vi "BLE_Sample - Test1.vi"() -> (2 "Table Control":string[][](table))   [LabVIEW 2020]
uses:
  C:/Users/bharathi.t/Downloads/Bluetooth - Copy/Bluetooth/BLE/BLELib.dll
  BLELib.dll
panel:
  out "DisConnect_BLE_ByAddress":bool
  out "ConnectionStatusChanged":string
  out "Numeric 2":i32
  out "error out":errorcluster
  out "Pair Result":string
  # "A4:DA:32:0D:F5:E2"
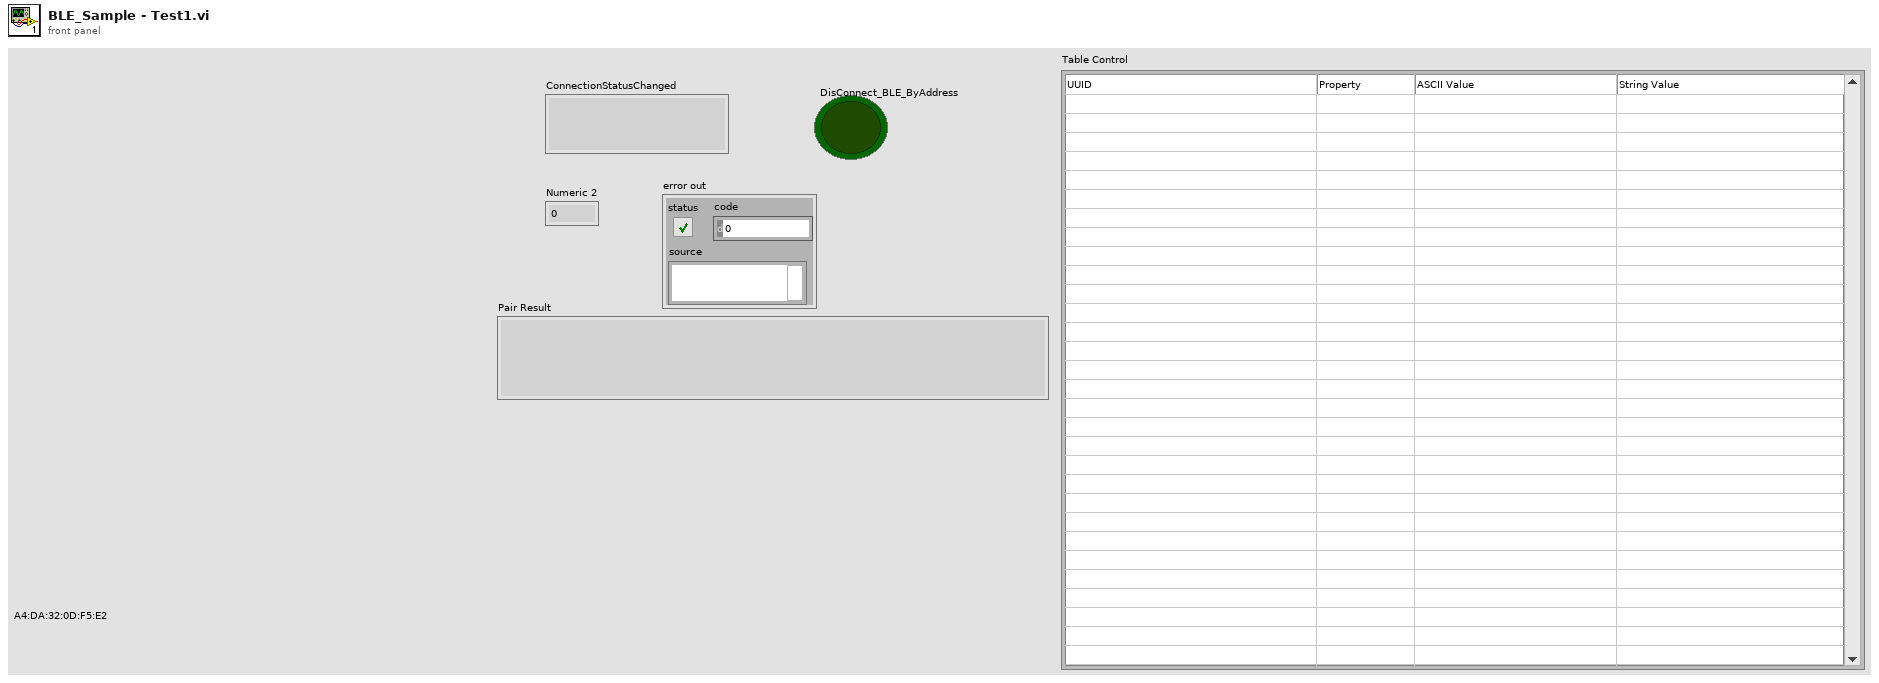
[diagram p1: front panel]
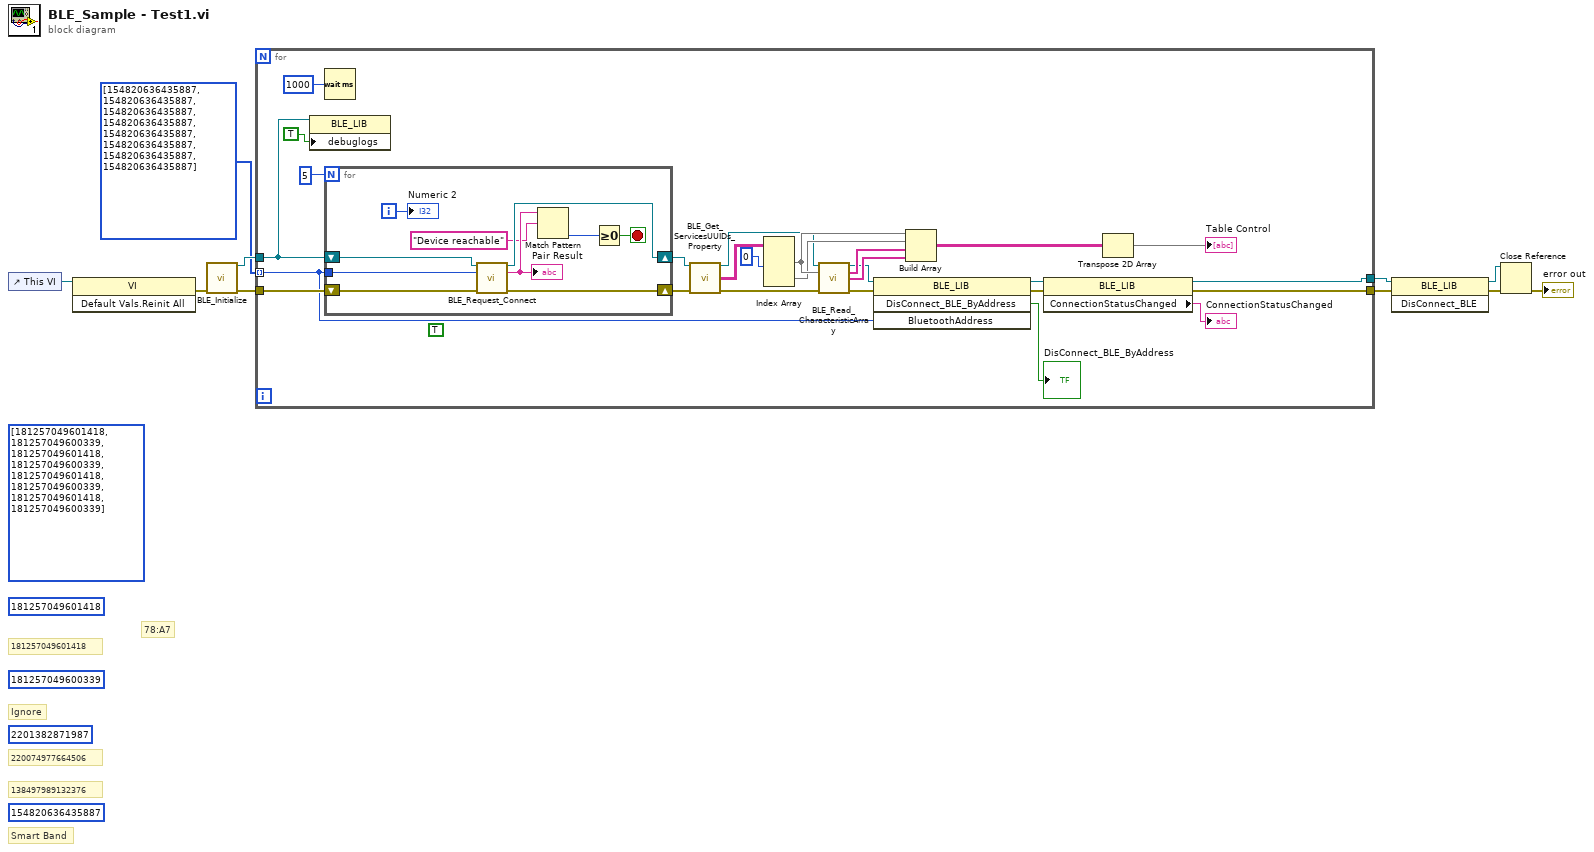
[diagram p0: block diagram]
diagram:
  (unwired) u64[] [181257049601418, 181257049600339, 181257049601418, 181257049600339, 181257049601418, 181257049600339, 181257049601418, 181257049600339]
  (unwired) u64 181257049600339 ("BluetoothAddress")
  (unwired) u64 2201382871987 ("BluetoothAddress")
  (unwired) u64 154820636435887 ("BluetoothAddress")
  (unwired) u64 181257049601418 ("BluetoothAddress")
  # "138497989132376"
  # "220074977664506"
  # "Ignore"
  # "78:A7"
  # "181257049601418"
  # "Smart Band"
  n1 = control-ref of="This VI"() -> (w10:refnum<vi>)
  n2 = invoke class="VI" method="Default Vals.Reinit All"(reference=w10) -> (error out=w8:errorcluster)  [unwired: 2 in, 2 out]
  n3 = call "BLE_Initialize.vi"("error in (no error)"=w8) -> (".NET Refnum out"=w6:refnum<k24>, "error out"=w7:errorcluster)  [unwired: 13 in]
  n4 = for {
    tunnel: [w14] -> w4
    tunnel: w6 -> [w21]
    tunnel: w7 -> [w20]
    tunnel: u64[] [154820636435887, 154820636435887, 154820636435887, 154820636435887, 154820636435887, 154820636435887, 154820636435887, 154820636435887] -> [w17] mode=indexing
    tunnel: [w15] -> w2
    (unwired) TRUE
    n5 = property class="BLE_LIB"(reference=w21, "debuglogs"=TRUE) -> ()  [unwired: 1 in, 2 out]
    n6 = Wait (ms)(milliseconds to wait=u32 1000) -> ()  [unwired: 1 out]
    n7 = for {
      N: 5 -> [_]
      tunnel: w17 -> [w44]
      shift-right: [w42] -> w34
      shift-left: w20 -> [w46]
      shift-right: [w43] -> w35
      shift-left: w21 -> [w45]
      i -> [w37]
      stop <- w38 stop-if-true
      n8 = call "BLE_Request_Connect.vi"(".NET Refnum in"=w45, "BluetoothAddress"=w44, "error in (no error)"=w46) -> (".NET Refnum out"=w43:refnum<k24>, "ConnectBLE"=w41:string, "error out"=w42:errorcluster)  [unwired: 10 in]
      "Pair Result" <- w41
      n9 = Match Pattern(string=w41, regular expression="Device reachable") -> (offset past match=w39:i32)  [unwired: 1 in, 3 out]
      n10 = Greater Or Equal To 0?(x=w39) -> (x >= 0?=w38:bool)
      "Numeric 2" <- w37
    }
    n11 = call "BLE_Get_ServicesUUIDs_Property.vi"(".NET Refnum in"=w35, "error in (no error)"=w34) -> (".NET Refnum out"=w23:refnum<k24>, "Char Val-Property"=w25:string[][], "error out"=w24:errorcluster)  [unwired: 11 in]
    n12 = Index Array(array=w25, index (col) #1=0 ("disabled index (col)")) -> (element #1=w28:string[], element #2=w27:string[])  [unwired: 3 in]
    n13 = call "BLE_Read_CharacteristicArray.vi"(".NET Refnum in"=w23, "ServicesUUIDs Extract Value"=w28, "error in (no error)"=w24) -> (".NET Refnum out"=w18:refnum<k24>, "ServicesUUIDs ASCII Value"=w32:string[], "ServicesUUIDs Value"=w31:string[], "error out"=w19:errorcluster)  [unwired: 9 in]
    n14 = invoke class="BLE_LIB" method="DisConnect_BLE_ByAddress"(reference=w18, error in=w19, "BluetoothAddress"=w17) -> (reference out=w16:refnum<k24>, error out=w12:errorcluster, "DisConnect_BLE_ByAddress"=→"DisConnect_BLE_ByAddress":bool)  [unwired: 1 in, 1 out]
    n15 = Build Array(w28, w27, w32, w31) -> (w30:string[][])
    n16 = property class="BLE_LIB"(reference=w16, error in=w12) -> (reference out=w14:refnum<k24>, error out=w15:errorcluster, "ConnectionStatusChanged"=→"ConnectionStatusChanged":string)
    n17 = Transpose 2D Array(2D array=w30) -> (transposed array=→"Table Control":string[][])
  }
  n18 = invoke class="BLE_LIB" method="DisConnect_BLE"(reference=w4, error in=w2) -> (reference out=w3:refnum<k24>, error out=w1:errorcluster)  [unwired: 1 in, 1 out]
  n19 = Close Reference(reference=w3, error in (no error)=w1) -> (error out=→"error out":errorcluster)
